vi "Waveform-Check For New.vi"(9 "Waveform names":string[](array[string]), 11 "State In":T1 caption="State") -> (3 "State Out":T1 caption="State")   [LabVIEW 2020, in "Waveform (G3).xctl"]
uses:
  Waveform (G3).xctl
  State.ctl
  Utility VIs/Controls/KRing/KRing.xctl
  Tone (G3)/Tone (G3).xctl
  Noise (G3)/Noise (G3).xctl
  Noise (G3)/Noise (G3) - Persistent.ctl
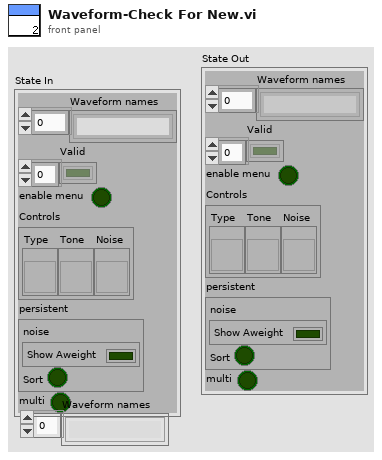
[diagram p1: front panel]
types:
  T1 = typedef "Waveform (G3).xctl/State.ctl" = cluster{"Waveform names":string[], "Valid":bool[], "enable menu":bool, "Controls":cluster{"Type ":refnum<vi>, "Tone ":refnum<vi>, "Noise":refnum<vi>}, "persistent":cluster{"noise":T2, "Sort":bool}, "multi":bool}
  T2 = typedef "Noise (G3).xctl/Noise (G3) - Persistent.ctl" = cluster{"Show Aweight":bool}
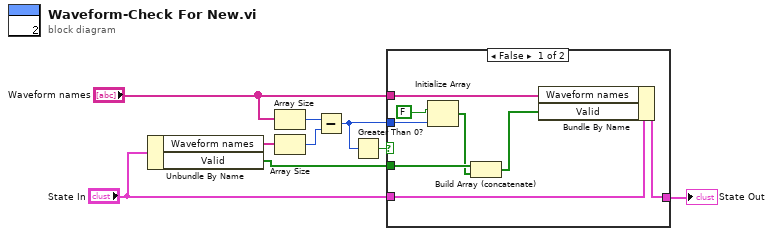
[diagram p0: block diagram]
diagram:
  n1 = Unbundle By Name("State In") -> ("Waveform names"=w2:string[], "Valid"=w8:bool[])
  n2 = Array Size(array="Waveform names") -> (size(s)=w5:i32)
  n3 = Array Size(array=w2) -> (size(s)=w6:i32)
  n4 = Subtract(x=w5, y=w6) -> (x-y=w9:i32)
  n5 = Greater Than 0?(x=w9) -> (x > 0?=w7:bool)
  n6 = case shown="False" w7 {
    tunnel: [w16 w18] -> w3
    tunnel: "State In" -> [w17 w18]
    tunnel: "Waveform names" -> [w15 _]
    tunnel: w8 -> [w13 _]
    tunnel: w9 -> [w11 _]
    frame False {
      n7 = Initialize Array(FALSE, w11) -> (w12:bool[])
      n8 = Build Array (concatenate)(w13, w12) -> (w10:bool[])
      n9 = Bundle By Name(cluster=w17, "Waveform names"=w15, "Valid"=w10) -> (w16:T1)
    }
    frame True {
    }
  }
  "State Out" <- w3
